vi "Th_timer.vi"   [LabVIEW 2018]
uses:
  Th_GUI.vi
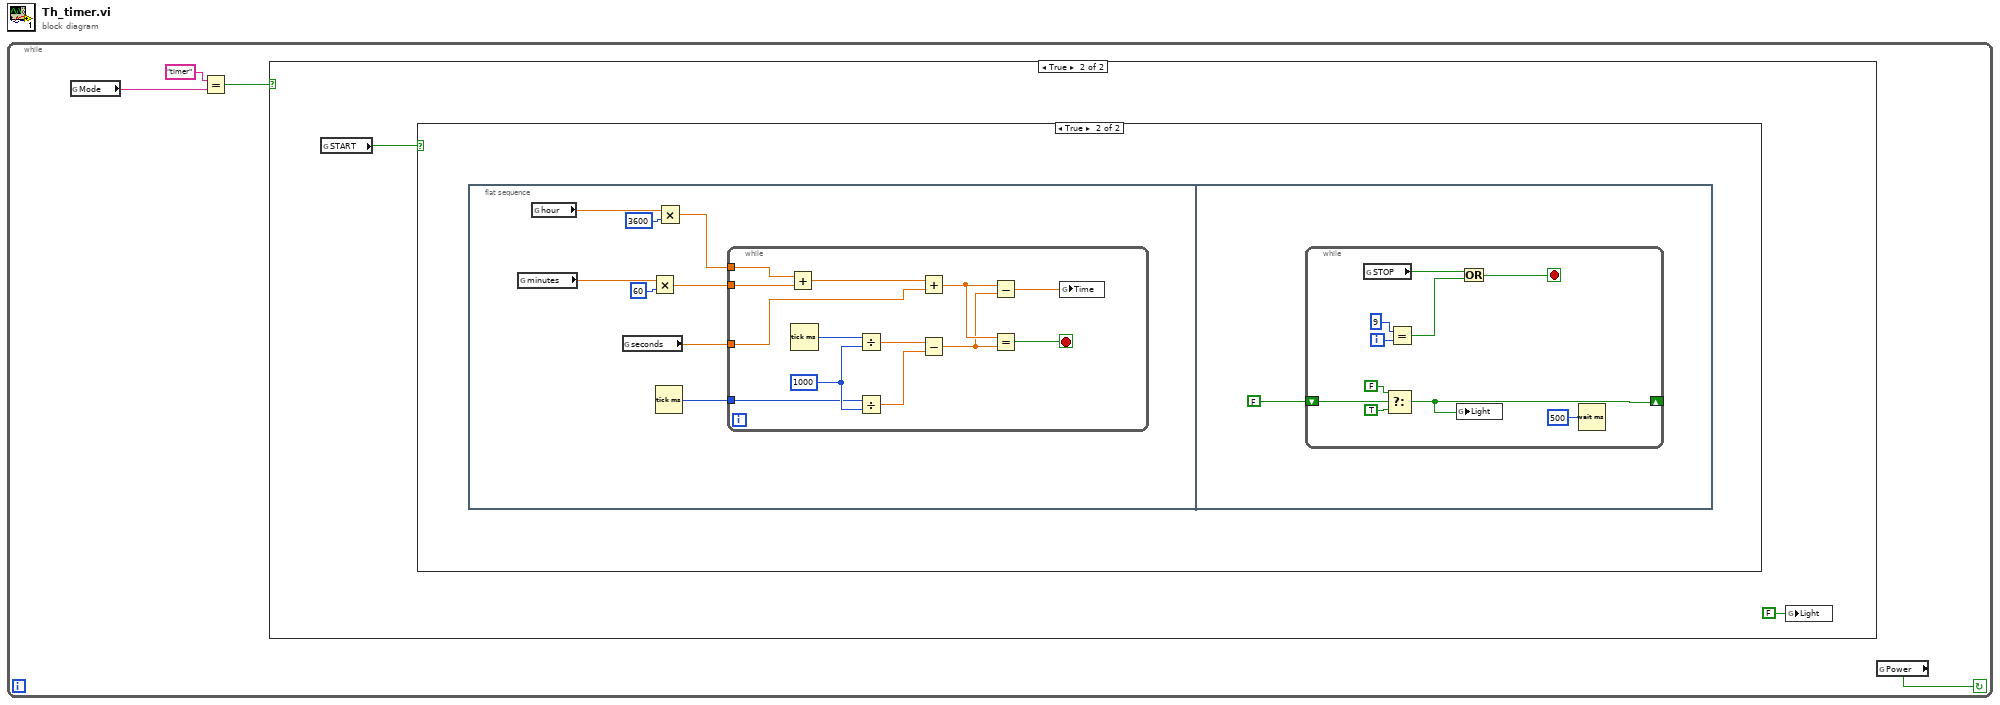
[diagram p0: block diagram]
diagram:
  n1 = while {
    stop <- w2 continue-if-true
    n2 = global read "Th_GUI.vi" "Mode"() -> (w3:string)
    n3 = Equal?(x="timer", y=w3) -> (x = y?=w1:bool)
    n4 = case shown="TRUE" w1 {
      frame False {
      }
      frame True {
        n5 = global read "Th_GUI.vi" "START"() -> (w6:bool)
        n6 = case shown="TRUE" w6 {
          frame False {
          }
          frame True {
            n7 = flat-sequence {
              frame #0 {
                n8 = global read "Th_GUI.vi" "minutes"() -> (w8:dbl)
                n9 = global read "Th_GUI.vi" "hour"() -> (w9:dbl)
                n10 = global read "Th_GUI.vi" "seconds"() -> (w7:dbl)
                n11 = Multiply(x=w8, y=60) -> (x*y=w12:dbl)
                n12 = Tick Count (ms)() -> (millisecond timer value=w10:u32)
                n13 = Multiply(x=w9, y=3600) -> (x*y=w11:dbl)
                n14 = while {
                  tunnel: w11 -> [w25]
                  tunnel: w12 -> [w24]
                  tunnel: w7 -> [w21]
                  tunnel: w10 -> [w16]
                  stop <- w23 stop-if-true
                  w19 = 1000
                  n15 = Add ("和")(x=w25, y=w24) -> (x+y=w22:dbl)
                  n16 = Tick Count (ms)() -> (millisecond timer value=w27:u32)
                  n17 = Divide(x=w27, y=w19) -> (x/y=w26:dbl)
                  n18 = Divide(x=w16, y=w19) -> (x/y=w20:dbl)
                  n19 = Add(x=w22, y=w21) -> (x+y=w18:dbl)
                  n20 = Subtract(x=w26, y=w20) -> (x-y=w17:dbl)
                  n21 = Subtract(x=w18, y=w17) -> (x-y=w15:dbl)
                  n22 = Equal?(x=w18, y=w17) -> (x = y?=w23:bool)
                  n23 = global write "Th_GUI.vi" "Time"(w15) -> ()
                }
              }
              frame #1 {
                n24 = while {
                  shift-right: [w34] -> _
                  shift-left: FALSE -> [w38]
                  i -> [w32]
                  stop <- w29 stop-if-true
                  n25 = global read "Th_GUI.vi" "STOP"() -> (w33:bool)
                  n26 = Select(t=FALSE, s=w38, f=TRUE) -> (s? t:f=w34:bool)
                  n27 = Equal?(x=9, y=w32) -> (x = y?=w30:bool)
                  n28 = global write "Th_GUI.vi" "Light"(w34) -> ()
                  n29 = Or(x=w33, y=w30) -> (x .or. y?=w29:bool)
                  n30 = Wait (ms)(milliseconds to wait=500) -> ()  [unwired: 1 out]
                }
              }
            }
          }
        }
        n31 = global write "Th_GUI.vi" "Light"(FALSE) -> ()
      }
    }
    n32 = global read "Th_GUI.vi" "Power"() -> (w2:bool)
  }
